vi "CoordinateConvert_CartesianToArm_Arrays.vi"(1 "XYPoints":T1[](array[typedef])) -> (0 "ArmCoordinates":T2[](array[typedef]))   [LabVIEW 2017]
uses:
  TypeDefs/ArmCoordinate.ctl
  General/PathPlanning/TypeDefs/Point2D.ctl
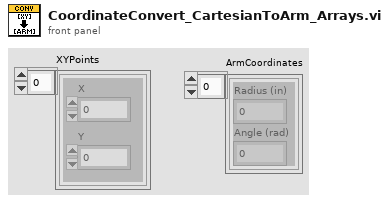
[diagram p1: front panel]
types:
  T1 = typedef "Point2D.ctl" = cluster{"X":dbl, "Y":dbl}
  T2 = typedef "ArmCoordinate.ctl" = cluster{"Radius (in)":dbl, "Angle (rad)":dbl}
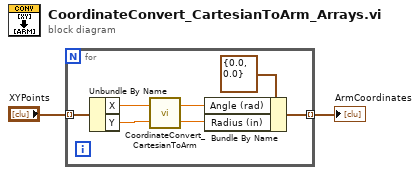
[diagram p0: block diagram]
diagram:
  n1 = for {
    tunnel: "XYPoints" -> [w9] mode=indexing
    tunnel: [w3] -> w1 mode=indexing
    n2 = Unbundle By Name(w9) -> ("X"=w8:dbl, "Y"=w7:dbl)
    n3 = call "CoordinateConvert_CartesianToArm.vi"("Y (in)"=w7, "X (in)"=w8) -> ("Radius (in)"=w5:dbl, "Angle (rad)"=w6:dbl)
    n4 = Bundle By Name(cluster=T2 {"Radius (in)"=0.0, "Angle (rad)"=0.0} ("Point"), "Angle (rad)"=w6, "Radius (in)"=w5) -> (w3:T2)
  }
  "ArmCoordinates" <- w1
